vi "Unit Test.vi"() -> ()   [LabVIEW 2018]
uses:
  GEN40-38-LAN.lvclass
  PPLs/Power Supply/Parent/Power_Supply.lvlibp/Custom Control/Supply Settings.ctl
  PPLs/Power Supply/Parent/Power_Supply.lvlibp/Custom Control/Protection.ctl
  PPLs/Power Supply/Parent/Power_Supply.lvlibp/Power Supply.lvclass
  PPLs/Power Supply/Parent/Power_Supply.lvlibp
  C:/Projects/LabVIEW/PPLs/Power Supply/Parent/Power_Supply.lvlibp/Power Supply.lvclass
panel:
  out "Alarm?":bool
  in  "Under Volt":dbl
  in  "Over Volt":dbl
  out "Output":bool
  in  "Settings":T1
  out "Current":dbl
  out "Voltage":dbl
  out "GEN40-38-LAN out":refnum<class "GEN40-38-LAN.lvclass">
  out "error out":errorcluster
  in  "error in":errorcluster
  in  "Resource":refnum<visa-resource-name>
  # "Unit Test VI:"
  # "1. Select Resource ID\n2. Provide input values for Voltage abd Current in the Settings cluster\n3. Provide Over Volt input value that is at least 1.05 times greater than the Voltage setting\n4. Provide Under Volt input value that is at least 0.95 times lower than the Voltage Setting\n5. Run the VI\n6. The VI will turn on the PS, for 2 seconds, take voltage, current, output  and alarm measurements.\n7. The VI will turn off the PS."
  # "TCPIP0::169.254.138.250::INSTR"
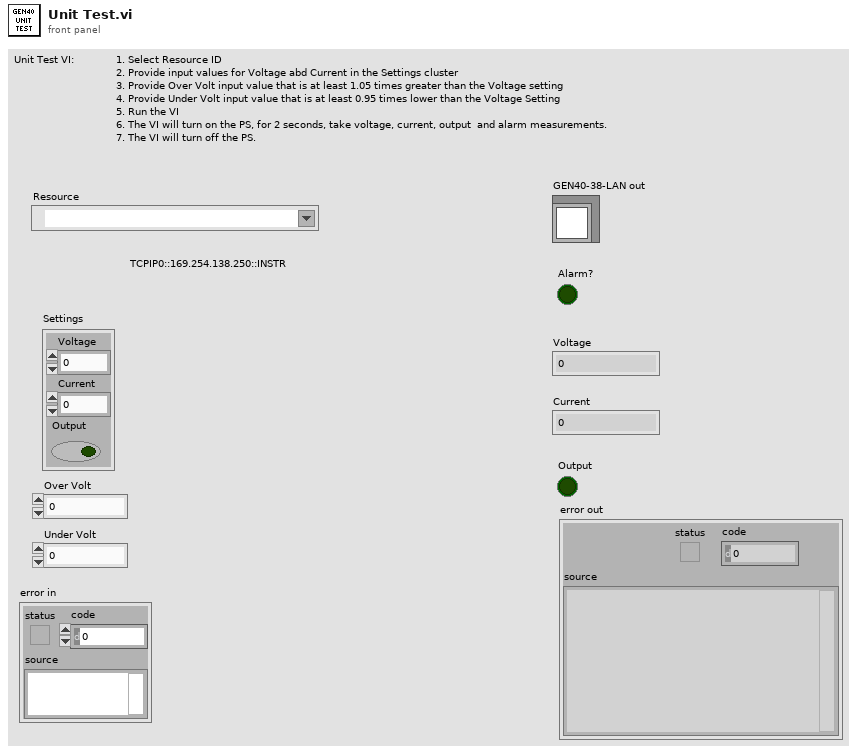
[diagram p1: front panel]
types:
  T1 = typedef "Power_Supply.lvlibp/Supply Settings.ctl" = cluster{"Voltage":dbl, "Current":dbl, "Output":bool}
  T2 = typedef "Power_Supply.lvlibp/Protection.ctl" = enum16{"None", "Over Volt", "Under Volt", "Over Current"}
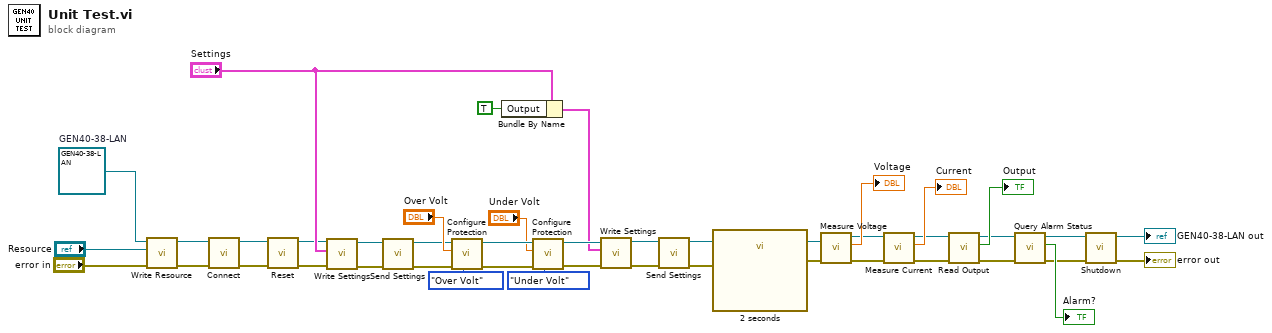
[diagram p0: block diagram]
diagram:
  w5 = refnum<class "GEN40-38-LAN.lvclass"> refnum  # GEN40-38-LAN
  n1 = call "Write Resource.vi"("error in"="error in", "Resource"="Resource", "Power Supply in"=w5) -> ("error out"=w41:errorcluster, "Power Supply out"=w40:refnum<class "GEN40-38-LAN.lvclass">)  [unwired: 7 in]
  n2 = call-dynamic "Connect.vi"("error in (no error)"=w41, "GEN40-38-LAN in"=w40) -> ("error out"=w8:errorcluster, "GEN40-38-LAN out"=w9:refnum<class "GEN40-38-LAN.lvclass">)  [unwired: 8 in]
  n3 = call-dynamic "Reset.vi"("error in (no error)"=w8, "GEN40-38-LAN in"=w9) -> ("error out"=w6:errorcluster, "GEN40-38-LAN out"=w7:refnum<class "GEN40-38-LAN.lvclass">)  [unwired: 8 in]
  n4 = call "Write Settings.vi"("error in (no error)"=w6, "Settings"="Settings", "Power Supply in"=w7) -> ("error out"=w19:errorcluster, "Power Supply out"=w20:refnum<class "GEN40-38-LAN.lvclass">)  [unwired: 7 in]
  n5 = call-dynamic "Send Settings.vi"("error in (no error)"=w19, "GEN40-38-LAN in"=w20) -> ("error out"=w18:errorcluster, "GEN40-38-LAN out"=w10:refnum<class "GEN40-38-LAN.lvclass">)  [unwired: 8 in]
  n6 = call-dynamic "Configure Protection.vi"("Protection (None)"=Protection."Over Volt", "error in (no error)"=w18, "Limit"="Over Volt", "GEN40-38-LAN in"=w10) -> ("error out"=w32:errorcluster, "GEN40-38-LAN out"=w31:refnum<class "GEN40-38-LAN.lvclass">)  [unwired: 6 in]
  n7 = Bundle By Name(cluster="Settings", "Output"=TRUE) -> (w12:T1)
  n8 = call-dynamic "Configure Protection.vi"("Protection (None)"=Protection."Under Volt", "error in (no error)"=w32, "Limit"="Under Volt", "GEN40-38-LAN in"=w31) -> ("error out"=w13:errorcluster, "GEN40-38-LAN out"=w14:refnum<class "GEN40-38-LAN.lvclass">)  [unwired: 6 in]
  n9 = call "Write Settings.vi"("error in (no error)"=w13, "Settings"=w12, "Power Supply in"=w14) -> ("error out"=w16:errorcluster, "Power Supply out"=w15:refnum<class "GEN40-38-LAN.lvclass">)  [unwired: 7 in]
  n10 = call-dynamic "Send Settings.vi"("error in (no error)"=w16, "GEN40-38-LAN in"=w15) -> ("error out"=w24:errorcluster, "GEN40-38-LAN out"=w25:refnum<class "GEN40-38-LAN.lvclass">)  [unwired: 8 in]
  n11 = call "2 seconds"("error in (no error)"=w24) -> ("error out"=w35:errorcluster)  [unwired: 10 in]
  n12 = call-dynamic "Measure Voltage.vi"("error in (no error)"=w35, "GEN40-38-LAN in"=w25) -> ("error out"=w37:errorcluster, "Voltage"=→"Voltage":dbl, "GEN40-38-LAN out"=w38:refnum<class "GEN40-38-LAN.lvclass">)  [unwired: 7 in]
  n13 = call-dynamic "Measure Current.vi"("error in (no error)"=w37, "GEN40-38-LAN in"=w38) -> ("error out"=w26:errorcluster, "Current"=→"Current":dbl, "GEN40-38-LAN out"=w34:refnum<class "GEN40-38-LAN.lvclass">)  [unwired: 7 in]
  n14 = call-dynamic "Read Output.vi"("error in"=w26, "GEN40-38-LAN in"=w34) -> ("error out"=w22:errorcluster, "Output"=→"Output":bool, "GEN40-38-LAN out"=w23:refnum<class "GEN40-38-LAN.lvclass">)  [unwired: 7 in]
  n15 = call-dynamic "Query Alarm Status.vi"("error in (no error)"=w22, "GEN40-38-LAN in"=w23) -> ("error out"=w2:errorcluster, "Alarm"=→"Alarm?":bool, "GEN40-38-LAN out"=w4:refnum<class "GEN40-38-LAN.lvclass">)  [unwired: 7 in]
  n16 = call "Shutdown.vi"("error in"=w2, "Power Supply in"=w4) -> ("error out"=→"error out":errorcluster, "Power Supply out"=→"GEN40-38-LAN out":refnum<class "GEN40-38-LAN.lvclass">)  [unwired: 8 in]
